vi "Get Open List.vi"(11 "AD* in":refnum<class "NI_Robotics_AnytimeDStar.lvclass">) -> (2 "Priority Queue":refnum<class "NI_Robotics_Priority Queue.lvclass">, 3 "AD* out":refnum<class "NI_Robotics_AnytimeDStar.lvclass">)   [LabVIEW 2017, in "NI_Robotics_AnytimeDStar.lvclass"]
uses:
  <vilib>/robotics/Navigation/Anytime D Star/NI_Robotics_AnytimeDStar.lvclass
  <vilib>/robotics/Navigation/shared/Priority Queue/NI_Robotics_Priority Queue.lvclass
  <vilib>/robotics/Navigation/Anytime D Star/NI_Robotics_AnytimeDStar.lvclass/NI_Robotics_AnytimeDStar.ctl
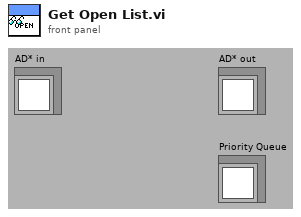
[diagram p1: front panel]
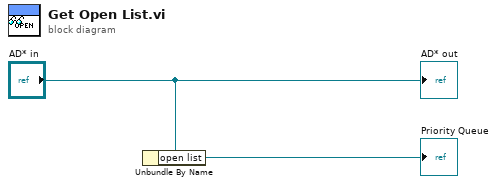
[diagram p0: block diagram]
diagram:
  n1 = Unbundle By Name("AD* in") -> ("open list"=→"Priority Queue":refnum<class "NI_Robotics_Priority Queue.lvclass">)
  "AD* out" <- "AD* in"
